vi "TCP Server Delete.vi"(8 "error in (no error)":errorcluster, 11 "TCP Server":refnum<class "JKI TCP Server.lvclass">) -> (0 "error out":errorcluster)   [LabVIEW 2020, in "JKI TCP Server.lvclass"]
uses:
  JKI TCP Server.lvclass
  JKI TCP Server.lvclass/JKI TCP Server.ctl
panel:
  # "OpenGOOP Delete.vi\n\nDestroys the GOOP object\n\nCopyright (C) 2002 Jim Kring jim@jimkring.com\n\nPlease visit http://www.OpenG.org to learn about the\nOpen Source LabVIEW software movement.\n\nThis library is free software; you can redistribute it and/or\nmodify it under the terms of the GNU Lesser General Public\nLicense as published by the Free Software Foundation; either\nversion 2.1 of the License, or (at your option) any later version.\nThis library is distributed in the hope that it will be useful,\nbut WITHOUT ANY WARRANTY; without even the implied warranty of\nMERCHANTABILITY or FITNESS FOR A PARTICULAR PURPOSE. See the GNU\nLesser General Public License for more details.\nYou should have received a copy of the GNU Lesser General Public\nLicense along with this library; if not, write to the Free Software\nFoundation, Inc., 59 Temple Place, Suite 330, Boston, MA 02111-1307 USA"
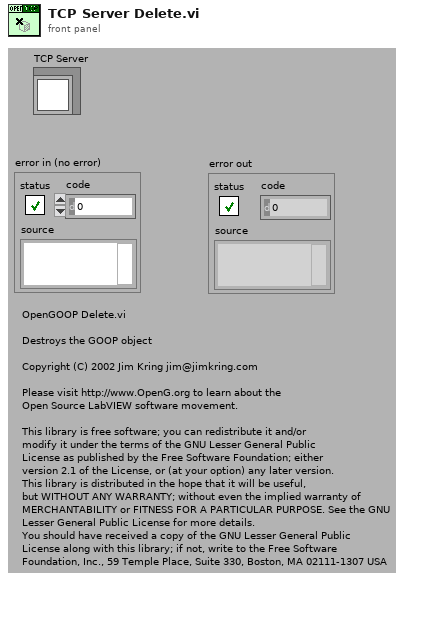
[diagram p1: front panel]
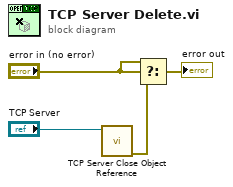
[diagram p0: block diagram]
diagram:
  n1 = call "TCP Server Close Object Reference.vi"("TCP Server"="TCP Server") -> ("error out"=w2:errorcluster)  [unwired: 10 in]
  n2 = Select(t="error in (no error)", s="error in (no error)", f=w2) -> (s? t:f=→"error out":errorcluster)
